vi "Set Transparent buttons.vi"(8 "error in":errorcluster, 10 "Transparent buttons?":bool, 11 "Plain Parent in":refnum<class "Plain Parent.lvclass">) -> (0 "error out":errorcluster, 3 "Plain Parent out":refnum<class "Plain Parent.lvclass">)   [LabVIEW 2021, in "Pop-Up.lvlib" / "Plain Parent.lvclass"]
doc: "DATA MEMBER ACCESS:\n\nSet the transparent button Boolean info"
uses:
  Plain Parent.lvclass
  Plain Parent.lvclass/Plain Parent.ctl
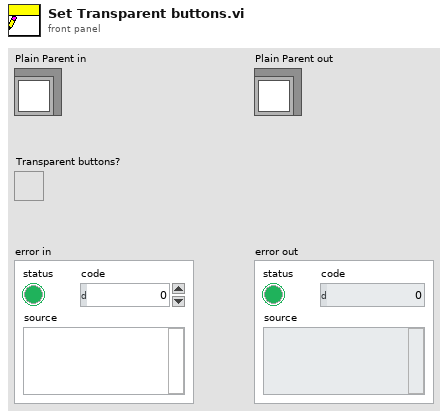
[diagram p1: front panel]
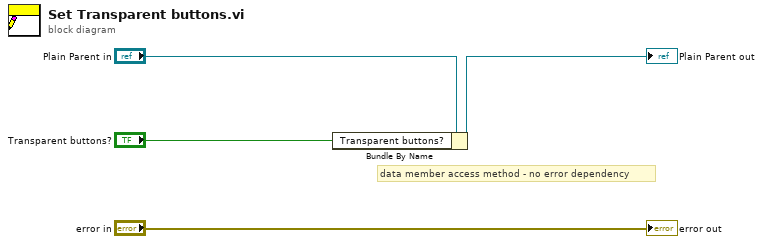
[diagram p0: block diagram]
diagram:
  # "data member access method - no error dependency"
  n1 = Bundle By Name(cluster="Plain Parent in", "Transparent buttons?"="Transparent buttons?") -> (→"Plain Parent out":refnum<class "Plain Parent.lvclass">)
  "error out" <- "error in"
